vi "Robot Move (with Controllers).vi"(9 "Reset":bool, 10 "Time Target":dbl=4.0 caption="Time Target (s)", 11 "Speed":dbl=-0.5 format="%#_13g") -> (3 "Stop?":bool)   [LabVIEW 2014]
uses:
  <vilib>/Rock Robotics/WPI/RobotDrive/WPI_RobotDriveGetSetRefNum.vi
  Robot Global Data.vi
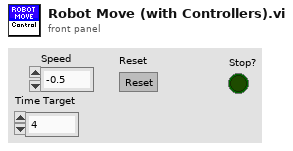
[diagram p1: front panel]
types:
  T1 = typedef "WPI_RobotDriveDevRef.ctl" = cluster{"DevStatus":errorcluster, "Motors[]":T2[], "Square Inputs":bool, "Max Output":dbl}
  T2 = typedef "WPI_MotorControlDeviceRef.ctl" = cluster{"DeviceStatus":errorcluster, "Type":T3, "PWM":cluster{"Controller":T4, "PWM Channel":T5, "DeadBand":T6}, "CAN":cluster{"Device Number":u8, "Control Mode":T7, "Semaphore":T8, "Max Vout":dbl, "TalonSRX Control Mode":T9}, "Invert":bool, "TransformRef":T10, "InvTransformRef":T10}
  T3 = typedef "WPI_MotorControlType.ctl" = enum16{"PWM", "CAN", "CANTalonSRX"}
  T4 = typedef "FPGA_TypedefDigitalModule.ctl" = enum16{"Controller 1"}
  T5 = typedef "FPGA_DIOPWMChannel.ctl" = enum8{"PWM 0", "PWM 1", "PWM 2", "PWM 3", "PWM 4", "PWM 5", "PWM 6", "PWM 7", "PWM 8", "PWM 9", "PWM MXP 0", "PWM MXP 1", "PWM MXP 2", "PWM MXP 3", "PWM MXP 4", "PWM MXP 5", "PWM MXP 6", "PWM MXP 7", "PWM MXP 8", "PWM MXP 9", "Invalid"}
  T6 = typedef "WPI_PWMDeadband.ctl" = cluster{"Name":string, "maxPositivePwm":i32, "minPositivePwm":i32, "centerPwm":i32, "maxNegativePwm":i32, "minNegativePwm":i32, "angularRange":u16}
  T7 = typedef "WPI_CANJaguar_ControlMode.ctl" = enum8{"Percent VBus", "Current", "Speed", "Position", "Voltage"}
  T8 = typedef "Semaphore RefNum" = refnum<k1>
  T9 = typedef "WPI_CANTalonSRX_APIControlMode.ctl" = enum8{"Percent VBus", "Speed", "Position", "Slave", "Unchanged / Invalid"}
  T10 = typedef "WPI_PWMTransform_ConPane.ctl" = refnum<vi>
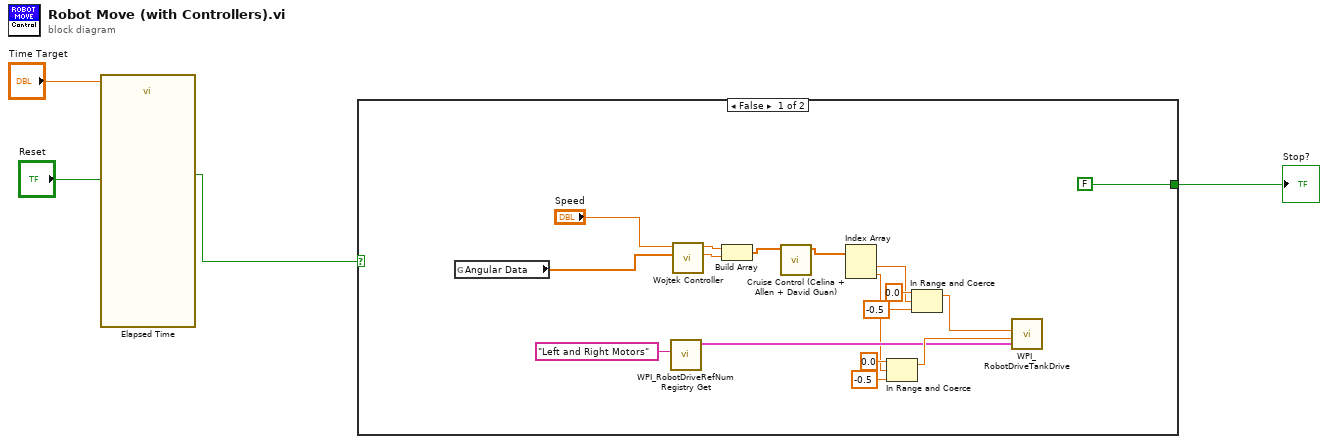
[diagram p0: block diagram]
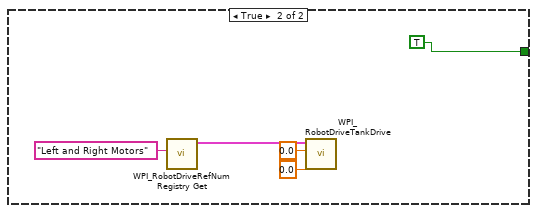
[diagram p2: hidden frame]
diagram:
  n1 = call "Elapsed Time"("Time Target (s)"="Time Target", "Reset"="Reset") -> ("Time has Elapsed"=w2:bool)  [unwired: 10 in, 7 out]
  n2 = case shown="False" w2 {
    tunnel: [FALSE TRUE] -> w4
    frame False {
      n3 = global read "Robot Global Data.vi" "Angular Data"() -> (w12:dbl[])
      n4 = call <vilib>:"WPI_RobotDriveRefNum Registry Get.vi"("refnum name"="Left and Right Motors") -> ("RobotDriveDevRef"=w13:T1)  [unwired: 1 in, 9 out]
      n5 = call "Wojtek Controller.vi"("Current Angle"=w12, "Speed"="Speed") -> ("left axis value"=w9:dbl, "right axis value"=w10:dbl)  [unwired: 8 in]
      n6 = Build Array(w10, w9) -> (w8:dbl[])
      n7 = call "Cruise Control (Celina + Allen + David Guan).vi"("Base Speed"=w8) -> ("output"=w11:dbl[])  [unwired: 10 in]
      n8 = Index Array(array=w11) -> (element #1=w7:dbl, element #2=w6:dbl)  [unwired: 2 in]
      n9 = In Range and Coerce(upper limit=0.0, x=w6, lower limit=-0.5) -> (coerced(x)=w21:dbl)  [unwired: 1 out]
      n10 = In Range and Coerce(upper limit=0.0, x=w7, lower limit=-0.5) -> (coerced(x)=w18:dbl)  [unwired: 1 out]
      n11 = call <vilib>:"WPI_RobotDriveTankDrive.vi"("Right axis value"=w21, "Left axis value"=w18, "RobotDriveDevRef"=w13) -> ()  [unwired: 6 in, 3 out]
    }
    frame True {
      n12 = call <vilib>:"WPI_RobotDriveRefNum Registry Get.vi"("refnum name"="Left and Right Motors") -> ("RobotDriveDevRef"=w26:T1)  [unwired: 9 in, 1 out]
      n13 = call <vilib>:"WPI_RobotDriveTankDrive.vi"("Right axis value"=0.0, "Left axis value"=0.0, "RobotDriveDevRef"=w26) -> ()  [unwired: 6 in, 3 out]
    }
  }
  "Stop?" <- w4
